vi "Test Waveform.vi"() -> ()   [LabVIEW 2016]
uses:
  <vilib>/xnet/xnet.llb/XNET Read (Signal Waveform) .vi
  <vilib>/xnet/xnet.llb/XNET Read (Signal Single-point).vi
  <vilib>/measure/NI_MAPro.lvlib
  <vilib>/measure/mamon.llb/Create Continuous Mask using Formula.vi
  <vilib>/measure/mamon.llb/Limit Testing Time.vi
panel:
  out "Y":dbl[](array[numeric])
  out "size(s)":i32
  out "Waveform Graph 3":cluster{"x0":dbl, "dx":dbl, "Y":dbl[]}(graph)
  out "element 2":waveform(dbl)
  out "Waveform Chart 3":waveform(dbl)[](graph)
  out "data 2":waveform(dbl)[](array[waveform]) caption="data"
  out "Waveform Graph 2":waveform(dbl)[](graph)
  out "Waveform Chart 2":waveform(dbl)[](graph)
  out "data":dbl[](array[numeric]) format="%.2f"
  in  "stop":bool
  out "Waveform Graph":waveform(dbl)(graph)
  out "Waveform Chart":waveform(dbl)(graph)
  out "element":dbl
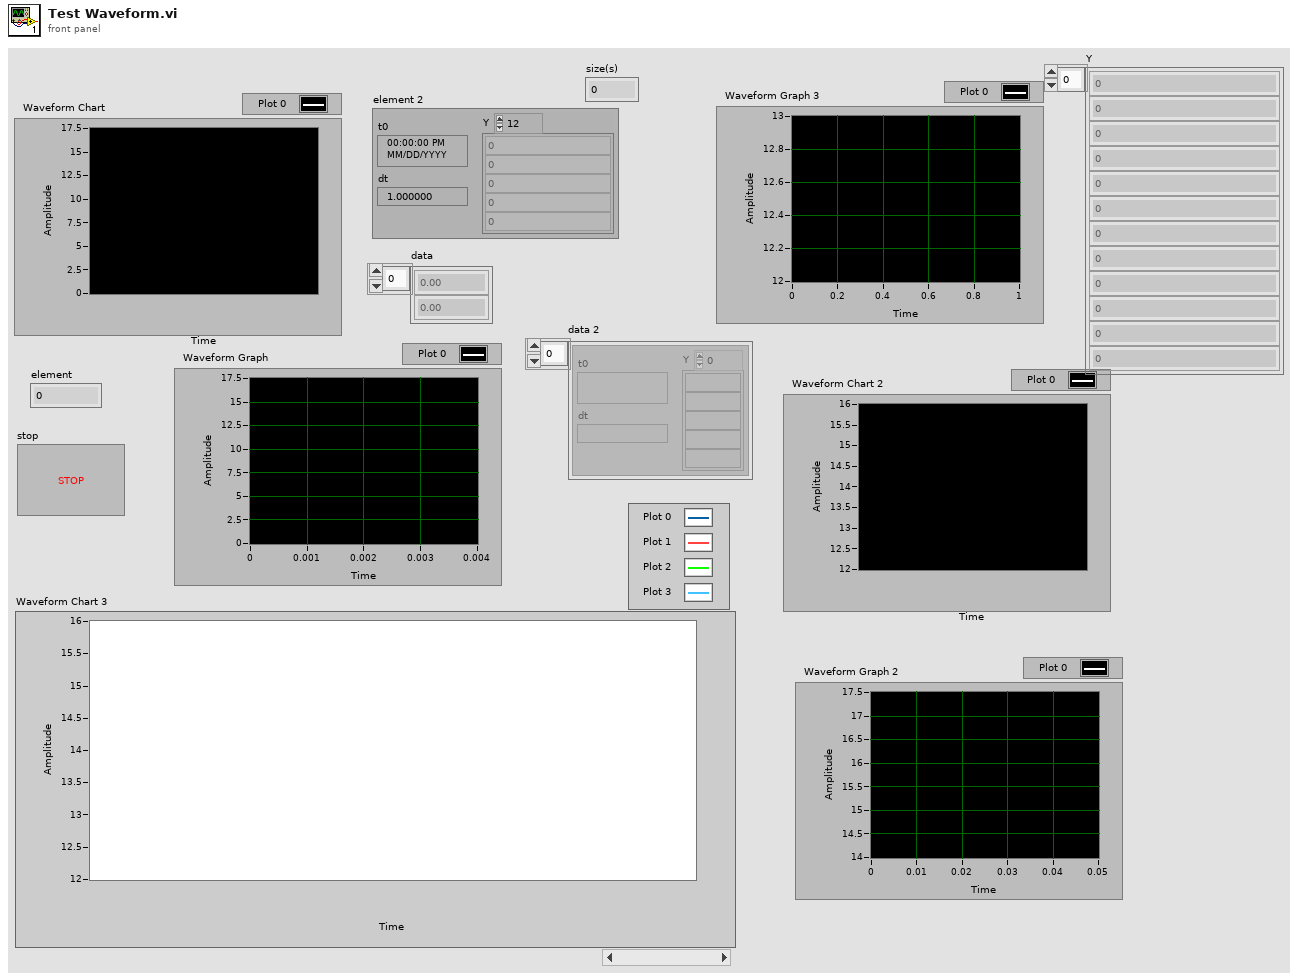
[diagram p1: front panel]
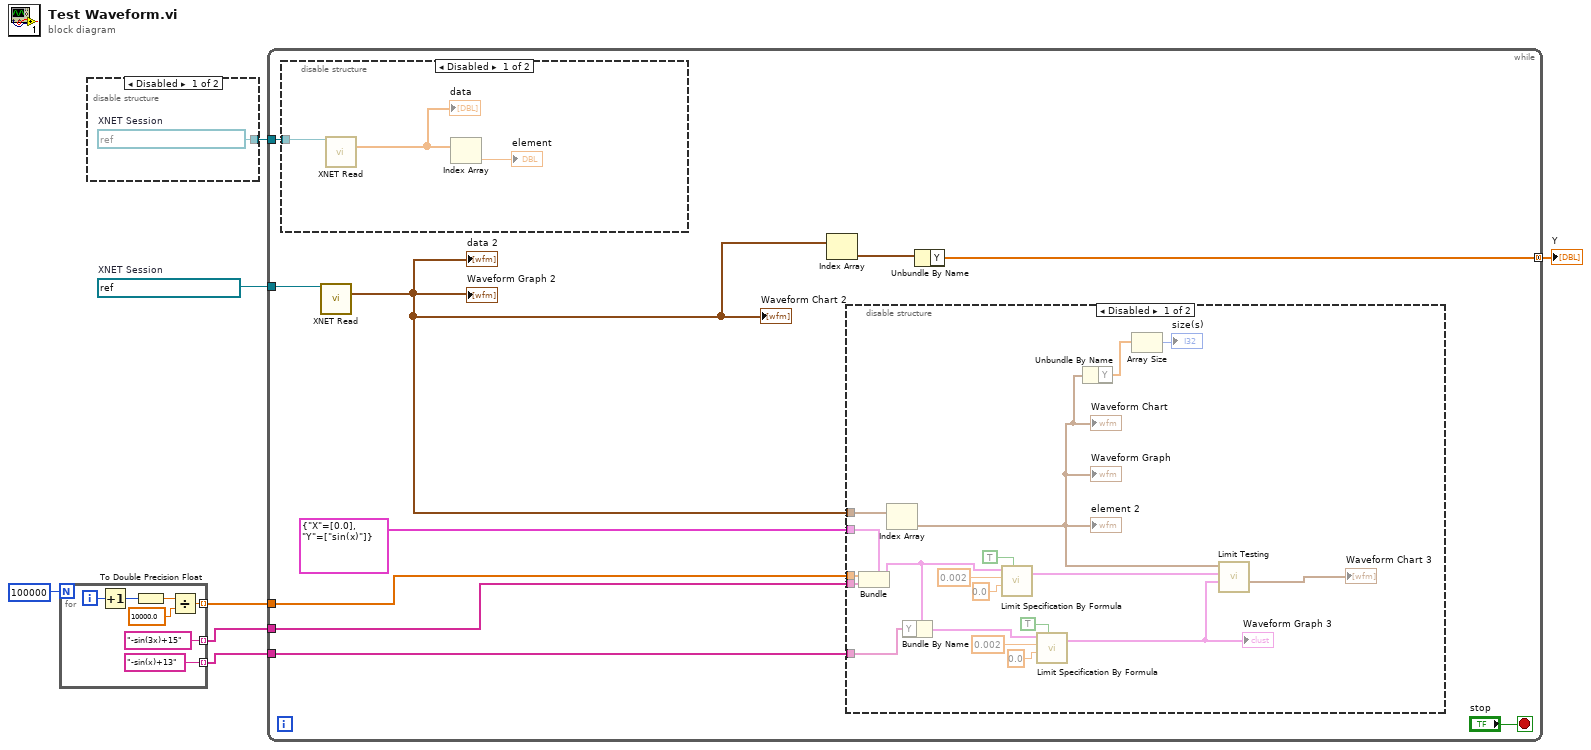
[diagram p0: block diagram]
diagram:
  w6 = refnum<k21> "New NI-XNET Session"  # XNET Session
  n1 = for {
    N: 100000 -> [_]
    tunnel: [w14] -> w4 mode=indexing
    tunnel: ["-sin(3x)+15" ("String")] -> w3 mode=indexing
    tunnel: ["-sin(x)+13" ("String")] -> w2 mode=indexing
    i -> [w11]
    n2 = Increment(x=w11) -> (x+1=w13:i32)
    n3 = To Double Precision Float(number=w13) -> (double precision float=w10:dbl)
    n4 = Divide(x=w10, y=10000.0) -> (x/y=w14:dbl)
  }
  n5 = disable-structure shown="Disabled" {
    disable-tunnel: [w15 _] -> w7
    frame Disabled {
      w15 = refnum<k21> "Analog In To CAN Ch1"  # XNET Session
    }
    frame Enabled {
    }
  }
  n6 = while {
    tunnel: w7 -> [w25]
    tunnel: w6 -> [w23]
    tunnel: w4 -> [w21]
    tunnel: w3 -> [w20]
    tunnel: w2 -> [w19]
    tunnel: [w16] -> w1 mode=concatenating
    stop <- "stop" stop-if-true
    n7 = disable-structure shown="Disabled" {
      disable-tunnel: w25 -> [w47 _]
      frame Disabled {
        n8 = call-poly <vilib>:"XNET Read.vi"("session in"=w47) -> ("data"=w45:dbl[])  [unwired: 12 in, 2 out]
        "data" <- w45
        n9 = Index Array(array=w45) -> (element=→"element":dbl)  [unwired: 1 in]
      }
      frame Enabled {
      }
    }
    n10 = call-poly <vilib>:"XNET Read.vi"("session in"=w23) -> ("data"=w18:waveform(dbl)[])  [unwired: 12 in, 2 out]
    "data 2" <- w18
    "Waveform Graph 2" <- w18
    "Waveform Chart 2" <- w18
    n11 = Index Array(array=w18) -> (element=w17:waveform(dbl))  [unwired: 1 in]
    n12 = disable-structure shown="Disabled" {
      disable-tunnel: cluster{"X":dbl[], "Y":string[]} {"X"=[0.0], "Y"=["sin(x)"]} ("Specification Cluster") -> [w37 _]
      disable-tunnel: w21 -> [w32 _]
      disable-tunnel: w20 -> [w31 _]
      disable-tunnel: w19 -> [w30 _]
      disable-tunnel: w18 -> [w29 _]
      frame Disabled {
        n13 = Bundle(cluster=w37, "X"=w32, "Y"=w31) -> (w43:cluster{"X":dbl[], "Y":string[]})
        n14 = Index Array(array=w29) -> (element=w28:waveform(dbl))  [unwired: 1 in]
        "Waveform Chart" <- w28
        "Waveform Graph" <- w28
        "element 2" <- w28
        n15 = Bundle By Name(cluster=w43, "Y"=w30) -> (w44:cluster{"X":dbl[], "Y":string[]})
        n16 = call-poly <vilib>:"Limit Specification By Formula.vi"("Specification Cluster"=w43, "dx"=0.002, "x0"=0.0, "Reset"=TRUE) -> ("Limit"=w40:cluster{"x0":dbl, "dx":dbl, "Y":dbl[]})  [unwired: 1 in, 1 out]
        n17 = call-poly <vilib>:"Limit Specification By Formula.vi"("Specification Cluster"=w44, "dx"=0.002, "x0"=0.0, "Reset"=TRUE) -> ("Limit"=w33:cluster{"x0":dbl, "dx":dbl, "Y":dbl[]})  [unwired: 1 in, 1 out]
        "Waveform Graph 3" <- w33
        n18 = Unbundle By Name(w28) -> ("Y"=w27:dbl[])
        n19 = Array Size(array=w27) -> (size(s)=→"size(s)":i32)
        n20 = call-poly <vilib>:"Limit Testing.vi"("lower limit"=w33, "upper limit"=w40, "signal in"=w28) -> ("output values"=→"Waveform Chart 3":waveform(dbl)[])  [unwired: 3 in, 5 out]
      }
      frame Enabled {
      }
    }
    n21 = Unbundle By Name(w17) -> ("Y"=w16:dbl[])
  }
  "Y" <- w1
